vi "acquireValue.vi"(8 "error in (no error)":errorcluster, 10 "nextSample?":bool, 11 "scbLink in":refnum<class "scbLink.lvclass">) -> (0 "error out":errorcluster, 1 "function return":i32, 2 "variantData":variant, 3 "scbLink out":refnum<class "scbLink.lvclass">)   [LabVIEW 2016, in "SALLV_AtDome_Messaging.lvlib" / "scbLink.lvclass"]
uses:
  scbLink.lvclass
  ts_sallv_AtDome/SALLV_AtDome.lvlib
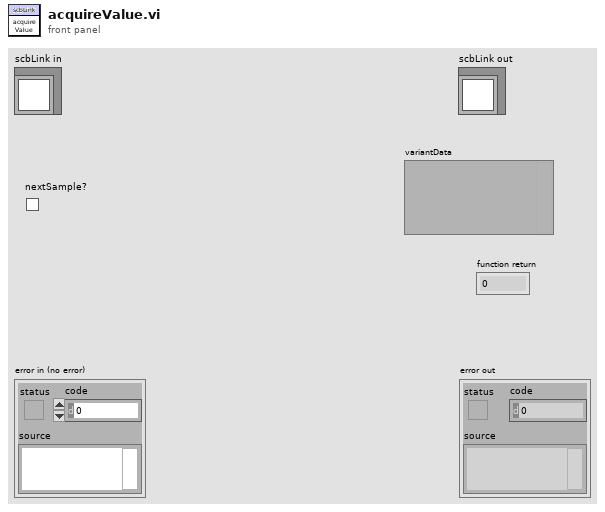
[diagram p1: front panel]
types:
  T1 = typedef "SALLV_AtDome.lvlib/logevent_scbLink.ctl" = cluster{"active":bool, "priority":i32}
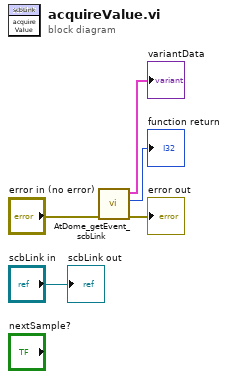
[diagram p0: block diagram]
diagram:
  n1 = call "AtDome_getEvent_scbLink.vi"("error in (no error)"="error in (no error)") -> ("error out"=→"error out":errorcluster, "function return"=→"function return":i32, "logevent_scbLink_Ctl out"=→"variantData":T1)  [unwired: 8 in]
  "scbLink out" <- "scbLink in"
